vi "Write Parameters.vi"(8 "error in (no error)":errorcluster, 10 "Mag Lab Parameters.lvclass":refnum<class "Mag Lab Parameters.lvclass">, 11 "Menu object array in":refnum<class "Menu object array.lvclass">) -> (0 "error out":errorcluster, 3 "Menu object array out":refnum<class "Menu object array.lvclass">)   [LabVIEW 2015, in "Menu object array.lvclass"]
uses:
  Menu object array.lvclass
  Mag Lab Properties/Mag Lab Parameters.lvclass
  Mag Lab Measure Interface/Mag Lab Measure UI.lvclass
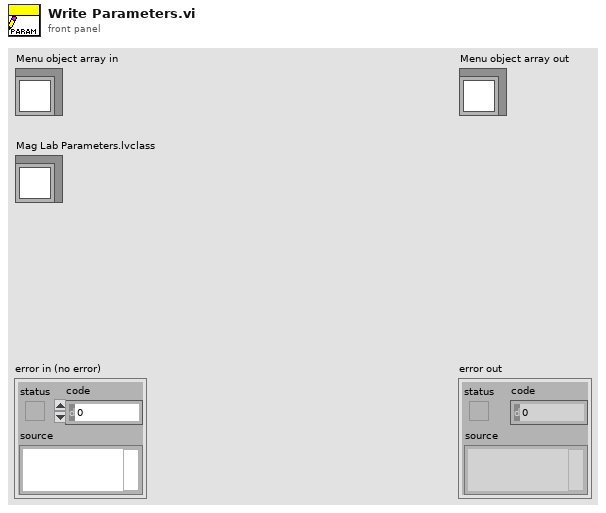
[diagram p1: front panel]
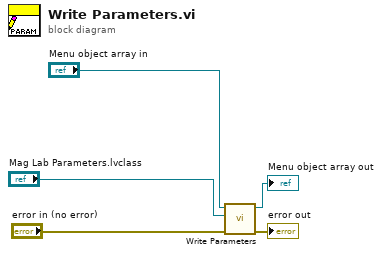
[diagram p0: block diagram]
diagram:
  n1 = call-parent "Write Parameters.vi"("error in (no error)"="error in (no error)", "Mag Lab Parameters.lvclass"="Mag Lab Parameters.lvclass", "Mag Lab Root in"="Menu object array in") -> ("error out"=→"error out":errorcluster, "Mag Lab Root out"=→"Menu object array out":refnum<class "Menu object array.lvclass">)  [unwired: 7 in]
